vi "Pixel Segments.vi"(8 "# px":i32, 9 "ds / px":dbl, 10 "End of First px":dbl, 11 "X":dbl[](array[numeric])) -> (2 "px Lengths":i32[](array[numeric]), 3 "px Starts":i32[](array[numeric]))   [LabVIEW 2020, in "VolatusGUIElements.lvlib"]
uses:
  VolatusGUIElements.lvlib
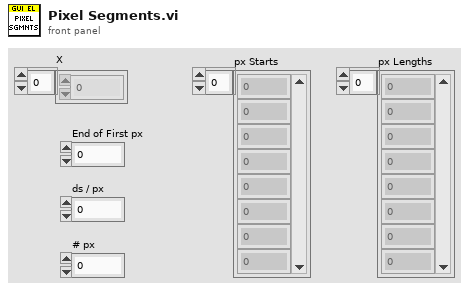
[diagram p1: front panel]
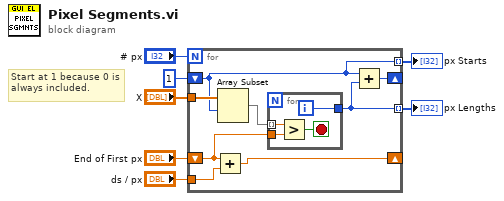
[diagram p0: block diagram]
diagram:
  # "Start at 1 because 0 is always included."
  n1 = for {
    N: "# px" -> [_]
    tunnel: "X" -> [w15]
    shift-right: [w14] -> _
    shift-left: 1 -> [w8]
    shift-right: [w12] -> _
    shift-left: "End of First px" -> [w10]
    tunnel: "ds / px" -> [w13]
    tunnel: [w9] -> w1 mode=indexing
    tunnel: [w8] -> w2 mode=indexing
    n2 = Add(x=w10, y=w13) -> (x+y=w12:dbl)
    n3 = Array Subset(array=w15, index=w8) -> (w11:dbl[])  [unwired: 1 in]
    n4 = for {
      tunnel: w11 -> [w19] mode=indexing
      tunnel: w10 -> [w18]
      tunnel: [w17] -> w9
      i -> [w17]
      stop <- w16 stop-if-true
      n5 = Greater?(x=w19, y=w18) -> (0:w16:bool)
    }
    n6 = Add(x=w8, y=w9) -> (x+y=w14:i32)
  }
  "px Starts" <- w2
  "px Lengths" <- w1
